vi "处理.vi"() -> ()   [LabVIEW 2014]
uses:
  F:/Program Files/labview2014/LABVIEW2014/examples/Instrument IO/Serial/support/Serial - Settings.ctl
  <vilib>/Instr/_visa.llb/VISA Configure Serial Port (Instr).vi
  <vilib>/httpClient/LabVIEWHTTPClient.lvlib
panel:
  out "result string 4":string
  out "result string 3":string
  in  "stop 3":bool
  in  "stop":bool
  in  "Serial Settings 2":T1={"baud rate"=9600, "data bits"=8, "parity"=enum."None", "stop bits"=10, "flow control"=0} {"flow control" items=["None"=0, "XON/XOFF"=1, "RTS/CTS"=2, "DTR/DSR"=4]; "stop bits" items=["1.0"=10, "1.5"=15, "2.0"=20]; "data bits" min=5 max=8 step=1; "baud rate" items=["75"=75, "110"=110, "134"=134, "150"=150, "300"=300, "600"=600, "1200"=1200, "1800"=1800, "2400"=2400, "4800"=4800, "7200"=7200, "9600"=9600, "14400"=14400, "19200"=19200, "28800"=28800, "38400"=38400, "56000"=56000, "57600"=57600, "115200"=115200, "128000"=128000, "230400"=230400]}
  in  "Serial Settings":T1={"baud rate"=9600, "data bits"=8, "parity"=enum."None", "stop bits"=10, "flow control"=0} {"flow control" items=["None"=0, "XON/XOFF"=1, "RTS/CTS"=2, "DTR/DSR"=4]; "stop bits" items=["1.0"=10, "1.5"=15, "2.0"=20]; "data bits" min=5 max=8 step=1; "baud rate" items=["75"=75, "110"=110, "134"=134, "150"=150, "300"=300, "600"=600, "1200"=1200, "1800"=1800, "2400"=2400, "4800"=4800, "7200"=7200, "9600"=9600, "14400"=14400, "19200"=19200, "28800"=28800, "38400"=38400, "56000"=56000, "57600"=57600, "115200"=115200, "128000"=128000, "230400"=230400]}
  out "result string 2":string
  out "return count 2":u32
  in  "stop 2":bool
  out "return count":u32
  out "result string":string
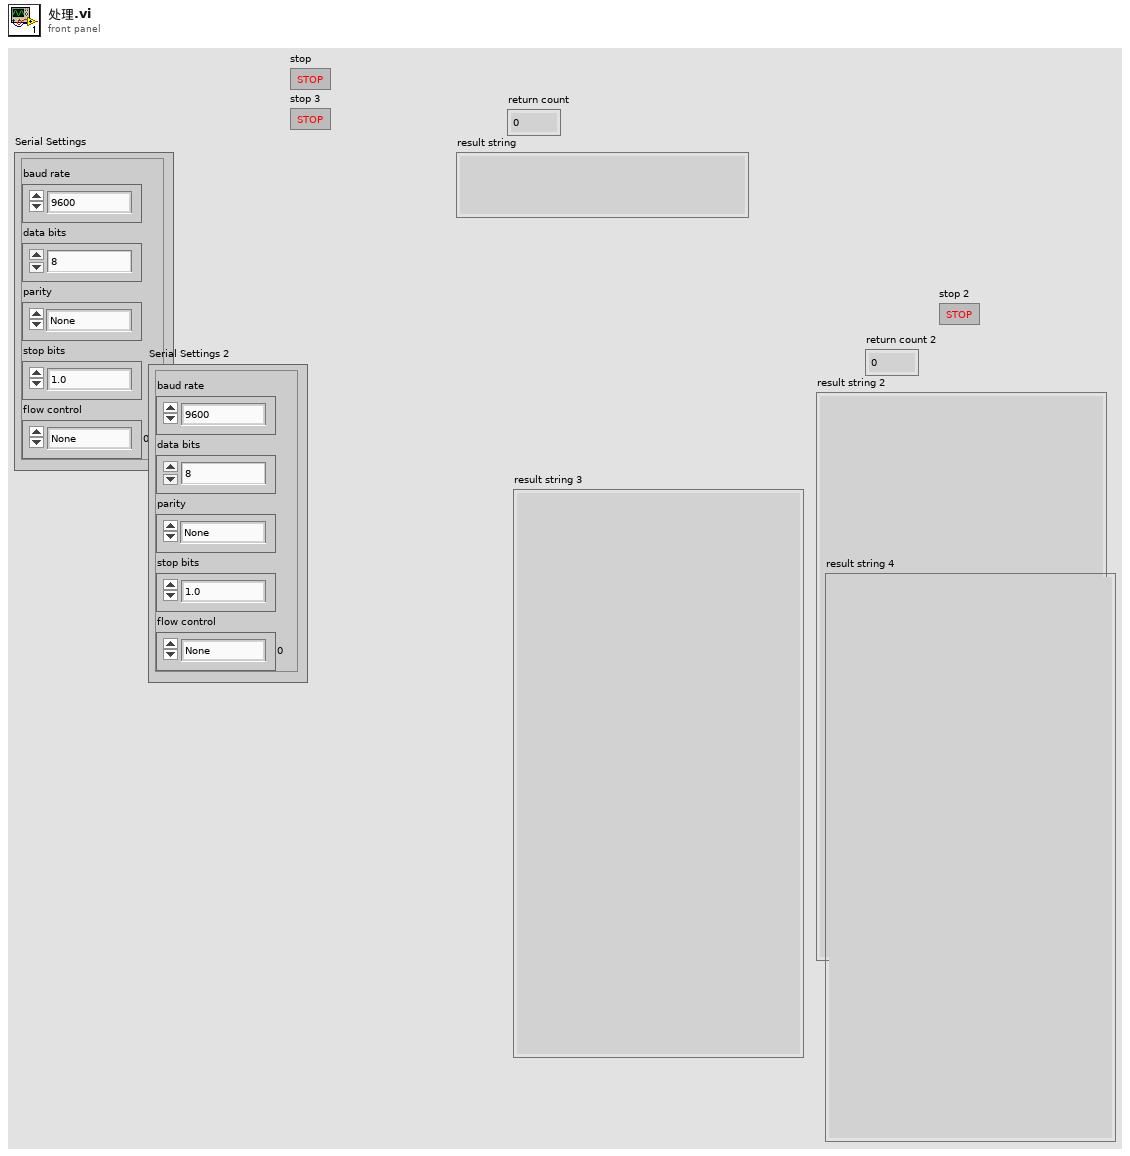
[diagram p1: front panel]
types:
  T1 = typedef "Serial - Settings.ctl" = cluster{"baud rate":u32, "data bits":u16, "parity":enum16{"None", "Odd", "Even", "Mark", "Space"}, "stop bits":u16, "flow control":u16}
  T2 = typedef "LabVIEWHTTPClient.lvlib/ClientHandle.ctl" = refnum<k1>
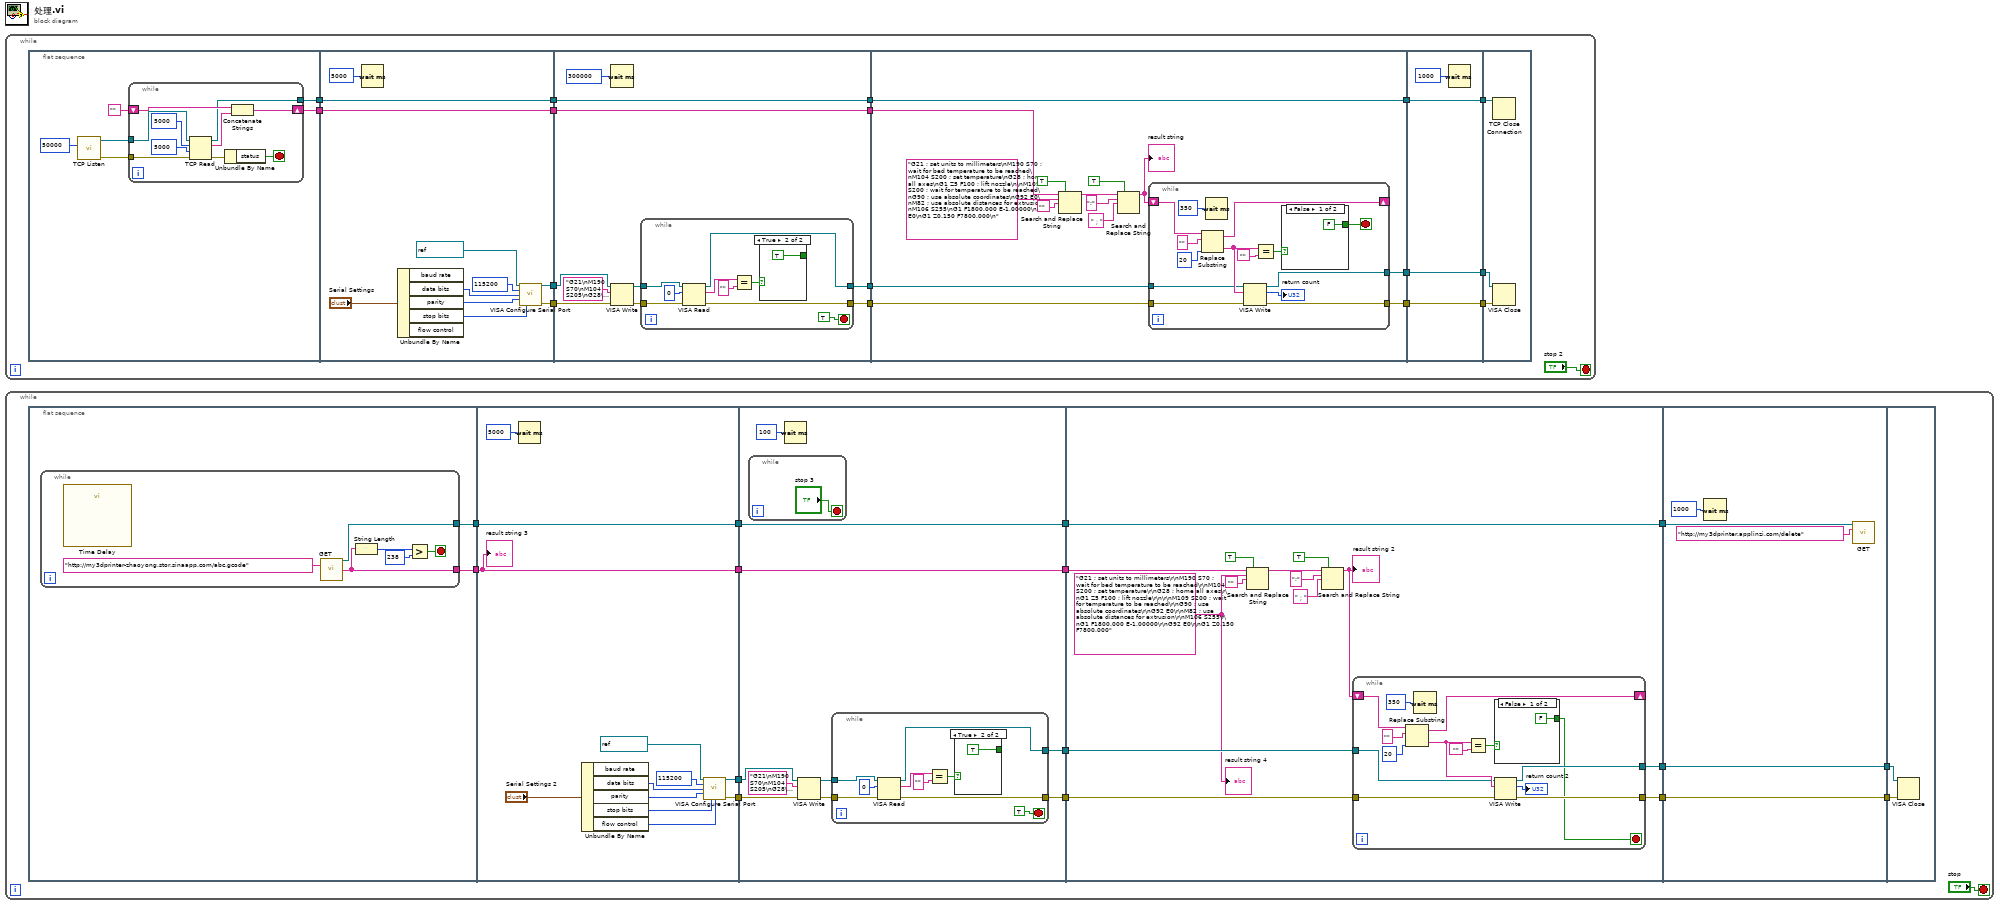
[diagram p0: block diagram]
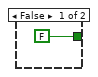
[diagram p2: hidden frame]
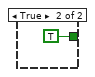
[diagram p3: hidden frame]
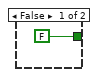
[diagram p4: hidden frame]
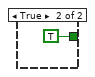
[diagram p5: hidden frame]
diagram:
  n1 = while {
    stop <- "stop 2" stop-if-true
    n2 = flat-sequence {
      tunnel: [w19] -> w4
      tunnel: [w18] -> w3
      tunnel: [w43] -> w8
      tunnel: [w42] -> w7
      tunnel: w4 -> [w43]
      tunnel: w3 -> [w42]
      tunnel: [w35] -> w2
      tunnel: [w34] -> w1
      tunnel: [w54] -> w17
      tunnel: [w53] -> w16
      tunnel: w8 -> [w54]
      tunnel: w7 -> [w53]
      tunnel: [w48] -> w6
      tunnel: [w47] -> w5
      tunnel: w2 -> [w46]
      tunnel: w1 -> [w45]
      tunnel: [w79] -> w15
      tunnel: [w78] -> w14
      tunnel: w17 -> [w69]
      tunnel: [w68] -> w13
      tunnel: w16 -> [w68]
      tunnel: w6 -> [w67]
      tunnel: w5 -> [w66]
      tunnel: w15 -> [w99]
      tunnel: [w99] -> w12
      tunnel: w14 -> [w98]
      tunnel: [w98] -> w11
      tunnel: w13 -> [w97]
      tunnel: [w97] -> w10
      tunnel: w12 -> [w102]
      tunnel: w11 -> [w101]
      tunnel: w10 -> [w100]
      frame #0 {
        n3 = call <vilib>:"TCP Listen.vi"("port"=u16 50000) -> ("error out"=w21:errorcluster, "connection ID"=w22:refnum<k5>)  [unwired: 6 in, 3 out]
        n4 = while {
          tunnel: w22 -> [w33]
          tunnel: w21 -> [w28]
          shift-right: [w31] -> w19
          shift-left: "" -> [w32]
          tunnel: [w30] -> w18
          stop <- w25 stop-if-true
          n5 = TCP Read(connection ID=w33, bytes to read=5000, error in (no error)=w28, 9:5000 ("timeout ms (25000)")) -> (connection ID out=w30:refnum<k5>, data out=w29:string, error out=w26:errorcluster)  [unwired: 1 in]
          n6 = Unbundle By Name(w26) -> ("status"=w25:bool)
          n7 = Concatenate Strings(w32, w29) -> (w31:string)
        }
      }
      frame #1 {
        n8 = Wait (ms)(milliseconds to wait=u32 5000) -> ()  [unwired: 1 out]
        n9 = Unbundle By Name("Serial Settings") -> ("data bits"=w41:u16, "parity"=w40:enum16{"None", "Odd", "Even", "Mark", "Space"}, "stop bits"=w39:u16)  [unwired: 2 out]
        n10 = call-poly "VISA Configure Serial Port"("VISA resource name"=refnum<visa-resource-name> "COM3", "baud rate (9600)"=u32 115200, "data bits (8)"=w41, "parity (0:none)"=w40, "stop bits (10: 1 bit)"=w39) -> ("VISA resource name out"=w35:refnum<visa-resource-name>, "error out"=w34:errorcluster)  [unwired: 5 in, 4 out]
      }
      frame #2 {
        n11 = Wait (ms)(milliseconds to wait=u32 300000) -> ()  [unwired: 1 out]
        n12 = VISA Write(VISA resource name=w46, write buffer="G21\nM190 S70\nM104 S205\nG28\nG1 Z5 F5000\nM109 S205\nG90\nG92 E0\nM82\nM106 S255\nG1 F1800.000 E-1.00000\nG92 E0\nG1 Z0.150 F7800.000\n", error in (no error)=w45) -> (VISA resource name out=w50:refnum<visa-resource-name>, error out=w51:errorcluster)  [unwired: 1 out]
        n13 = while {
          tunnel: w50 -> [w63]
          tunnel: [w62] -> w48
          tunnel: [w61] -> w47
          tunnel: w51 -> [w58]
          stop <- TRUE stop-if-true
          n14 = VISA Read(VISA resource name=w63, byte count=u32 0, error in (no error)=w58) -> (VISA resource name out=w62:refnum<visa-resource-name>, read buffer=w59:string, error out=w61:errorcluster)  [unwired: 1 out]
          n15 = Equal?(x=w59, y="") -> (x = y?=w60:bool)
          n16 = case shown="True" w60 {
            tunnel: [FALSE TRUE] -> _
            frame False {
            }
            frame True {
            }
          }
        }
      }
      frame #3 {
        n17 = Search and Replace String(replace all?=TRUE ("replace all? (F)"), input string=w69, search string="G21 ; set units to millimeters\nM190 S70 ; wait for bed temperature to be reached\nM104 S200 ; set temperature\nG28 ; home all axes\nG1 Z5 F100 ; lift nozzle\n\nM109 S200 ; wait for temperature to be reached\nG90 ; use absolute coordinates\nG92 E0\nM82 ; use absolute distances for extrusion\nM106 S255\nG1 F1800.000 E-1.00000\nG92 E0\nG1 Z0.150 F7800.000\n", replace string="") -> (result string=w72:string)  [unwired: 4 in, 3 out]
        n18 = Search and Replace String(replace all?=TRUE ("replace all? (F)"), input string=w72, search string=";", replace string="；" ("replace string (\"\")")) -> (result string=w70:string)  [unwired: 4 in, 3 out]
        "result string" <- w70
        n19 = while {
          shift-right: [w90] -> _
          shift-left: w70 -> [w91]
          tunnel: [w88] -> w79
          tunnel: [w87] -> w78
          tunnel: w67 -> [w82]
          tunnel: w66 -> [w81]
          stop <- w80 stop-if-true
          n20 = Replace Substring(2:20 ("length (len. of substring)"), 4:"" ("substring (\"\")"), 5:w91) -> (0:w84:string, 1:w90:string)  [unwired: 1 in]
          n21 = Wait (ms)(milliseconds to wait=u32 350) -> ()  [unwired: 1 out]
          n22 = VISA Write(VISA resource name=w82, write buffer=w84, error in (no error)=w81) -> (VISA resource name out=w87:refnum<visa-resource-name>, return count=→"return count":u32, error out=w88:errorcluster)
          n23 = Equal?(x=w84, y="") -> (x = y?=w86:bool)
          n24 = case shown="False" w86 {
            tunnel: [FALSE TRUE] -> w80
            frame False {
            }
            frame True {
            }
          }
        }
      }
      frame #4 {
        n25 = Wait (ms)(milliseconds to wait=u32 1000) -> ()  [unwired: 1 out]
      }
      frame #5 {
        n26 = TCP Close Connection(connection ID=w100) -> ()  [unwired: 2 in, 2 out]
        n27 = VISA Close(VISA resource name=w101, error in (no error)=w102) -> ()  [unwired: 1 out]
      }
    }
  }
  n28 = while {
    stop <- "stop" stop-if-true
    n29 = flat-sequence {
      tunnel: [w120] -> w118
      tunnel: [w119] -> w103
      tunnel: [w131] -> w117
      tunnel: [w130] -> w116
      tunnel: [w127] -> w115
      tunnel: w118 -> [w127]
      tunnel: [w128] -> w104
      tunnel: w103 -> [w128]
      tunnel: [w145] -> w114
      tunnel: [w144] -> w113
      tunnel: w117 -> [w142]
      tunnel: w116 -> [w143]
      tunnel: w115 -> [w141]
      tunnel: [w141] -> w112
      tunnel: [w139] -> w105
      tunnel: w104 -> [w139]
      tunnel: [w167] -> w111
      tunnel: [w166] -> w110
      tunnel: w114 -> [w165]
      tunnel: w113 -> [w164]
      tunnel: w112 -> [w163]
      tunnel: [w162] -> w106
      tunnel: w105 -> [w162]
      tunnel: [w194] -> w109
      tunnel: w111 -> [w194]
      tunnel: w110 -> [w193]
      tunnel: [w193] -> w108
      tunnel: w106 -> [w192]
      tunnel: w109 -> [w197]
      tunnel: w108 -> [w196]
      frame #0 {
        n30 = while {
          tunnel: [w122] -> w120
          tunnel: [w121] -> w119
          stop <- w123 stop-if-true
          n31 = call "Time Delay"() -> ()  [unwired: 11 in, 1 out]
          n32 = call <vilib>:"GET.vi"("url"="http://my3dprinter-zhaoyong.stor.sinaapp.com/abc.gcode") -> ("client handle out"=w121:T2, "body"=w122:string)  [unwired: 11 in, 2 out]
          n33 = String Length(string=w122) -> (length=w125:i32)
          n34 = Greater?(x=w125, y=238) -> (0:w123:bool)
        }
      }
      frame #1 {
        n35 = Wait (ms)(milliseconds to wait=u32 5000) -> ()  [unwired: 1 out]
        n36 = Unbundle By Name("Serial Settings 2") -> ("data bits"=w137:u16, "parity"=w136:enum16{"None", "Odd", "Even", "Mark", "Space"}, "stop bits"=w135:u16, "flow control"=w138:u16)  [unwired: 1 out]
        n37 = call-poly "VISA Configure Serial Port"("VISA resource name"=refnum<visa-resource-name> "COM3", "baud rate (9600)"=u32 115200, "data bits (8)"=w137, "parity (0:none)"=w136, "stop bits (10: 1 bit)"=w135, "flow control (0:none)"=w138) -> ("VISA resource name out"=w131:refnum<visa-resource-name>, "error out"=w130:errorcluster)  [unwired: 4 in, 4 out]
        "result string 3" <- w127
      }
      frame #2 {
        n38 = while {
          stop <- "stop 3" stop-if-true
        }
        n39 = Wait (ms)(milliseconds to wait=u32 100) -> ()  [unwired: 1 out]
        n40 = VISA Write(VISA resource name=w142, write buffer="G21\nM190 S70\nM104 S205\nG28\nG1 Z5 F5000\nM109 S205\nG90\nG92 E0\nM82\nM106 S255\nG1 F1800.000 E-1.00000\nG92 E0\nG1 Z0.150 F7800.000\n", error in (no error)=w143) -> (VISA resource name out=w147:refnum<visa-resource-name>, error out=w148:errorcluster)  [unwired: 1 out]
        n41 = while {
          tunnel: w147 -> [w158]
          tunnel: [w157] -> w144
          tunnel: [w156] -> w145
          tunnel: w148 -> [w153]
          stop <- TRUE stop-if-true
          n42 = VISA Read(VISA resource name=w158, byte count=u32 0, error in (no error)=w153) -> (VISA resource name out=w157:refnum<visa-resource-name>, read buffer=w154:string, error out=w156:errorcluster)  [unwired: 1 out]
          n43 = Equal?(x=w154, y="") -> (x = y?=w155:bool)
          n44 = case shown="True" w155 {
            tunnel: [FALSE TRUE] -> _
            frame False {
            }
            frame True {
            }
          }
        }
      }
      frame #3 {
        w161 = "G21 ; set units to millimeters\r\nM190 S70 ; wait for bed temperature to be reached\r\nM104 S200 ; set temperature\r\nG28 ; home all axes\r\nG1 Z5 F100 ; lift nozzle\r\n\r\nM109 S200 ; wait for temperature to be reached\r\nG90 ; use absolute coordinates\r\nG92 E0\r\nM82 ; use absolute distances for extrusion\r\nM106 S255\r\nG1 F1800.000 E-1.00000\r\nG92 E0\r\nG1 Z0.150 F7800.000" ("search string")
        n45 = Search and Replace String(replace all?=TRUE ("replace all? (F)"), input string=w163, search string=w161, replace string="") -> (result string=w170:string)  [unwired: 4 in, 3 out]
        n46 = Search and Replace String(replace all?=TRUE ("replace all? (F)"), input string=w170, search string=";", replace string="；" ("replace string (\"\")")) -> (result string=w168:string)  [unwired: 4 in, 3 out]
        "result string 2" <- w168
        n47 = while {
          shift-right: [w185] -> _
          shift-left: w168 -> [w186]
          tunnel: [w183] -> w166
          tunnel: [w182] -> w167
          tunnel: w165 -> [w177]
          tunnel: w164 -> [w176]
          stop <- w175 stop-if-true
          n48 = Replace Substring(2:20 ("length (len. of substring)"), 4:"" ("substring (\"\")"), 5:w186) -> (0:w179:string, 1:w185:string)  [unwired: 1 in]
          n49 = Wait (ms)(milliseconds to wait=u32 350) -> ()  [unwired: 1 out]
          n50 = Equal?(x=w179, y="") -> (x = y?=w181:bool)
          n51 = case shown="False" w181 {
            tunnel: [FALSE TRUE] -> w175
            frame False {
            }
            frame True {
            }
          }
          n52 = VISA Write(VISA resource name=w176, write buffer=w179, error in (no error)=w177) -> (VISA resource name out=w182:refnum<visa-resource-name>, return count=→"return count 2":u32, error out=w183:errorcluster)
        }
        "result string 4" <- w161
      }
      frame #4 {
        n53 = Wait (ms)(milliseconds to wait=u32 1000) -> ()  [unwired: 1 out]
        n54 = call <vilib>:"GET.vi"("client handle"=w192, "url"="http://my3dprinter.applinzi.com/delete") -> ()  [unwired: 10 in, 4 out]
      }
      frame #5 {
        n55 = VISA Close(VISA resource name=w197, error in (no error)=w196) -> ()  [unwired: 1 out]
      }
    }
  }
